vi "BEditor-PopoulateVIHelp.vi"(7 "Reference":variant, 8 "Error in":errorcluster caption="Error in (no error)", 9 "Option":variant, 11 "Entry":string) -> (0 "Error out":errorcluster)   [LabVIEW 2017, in "csmdoc.lvlib"]
uses:
  _Typedef/DocElement.ctl
  csmdoc.lvlib
  Communicable State Machine.lvlib
  _Shared/CSM Shared.lvlib
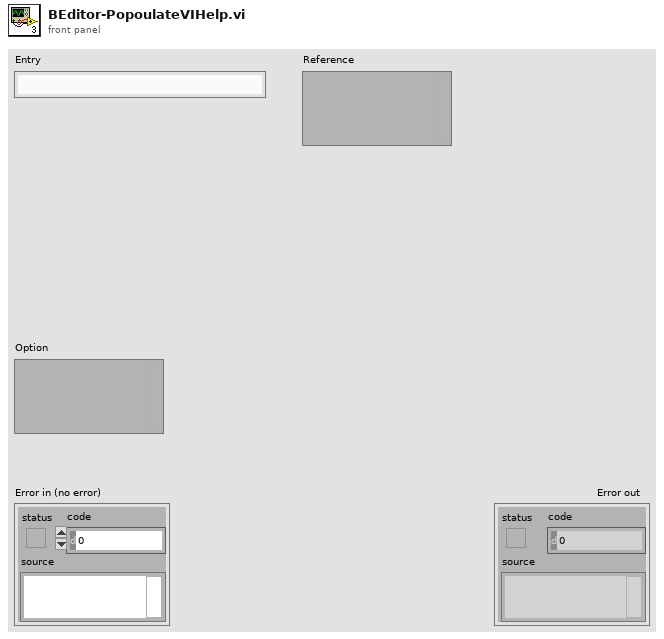
[diagram p1: front panel]
types:
  T1 = typedef "csmdoc.lvlib/DocElement.ctl" = cluster{"ID":string, "Content":string[], "SubIDs":string[], "Path":string[]}
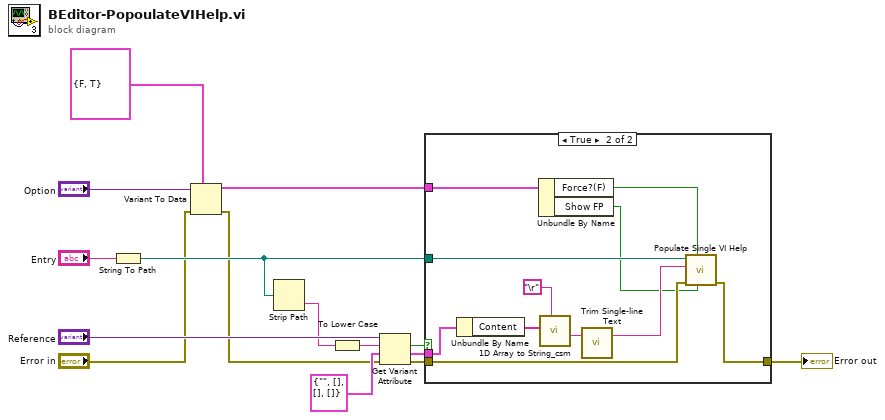
[diagram p0: block diagram]
diagram:
  n1 = String To Path(string="Entry") -> (path=w6:path)
  n2 = Variant To Data(error in="Error in", type=cluster{"Force?(F)":bool, "Show FP":bool} {"Force?(F)"=FALSE, "Show FP"=TRUE}, Variant="Option") -> (data=w1:cluster{"Force?(F)":bool, "Show FP":bool}, error out=w2:errorcluster)
  n3 = Strip Path(path=w6) -> (name=w13:string)  [unwired: 1 out]
  n4 = To Lower Case(string=w13) -> (all lower case string=w9:string)
  n5 = Get Variant Attribute(Variant="Reference", name=w9, default value (empty Variant)=T1 {"ID"="", "Content"=[], "SubIDs"=[], "Path"=[]} ("Cluster"), error in=w2) -> (found=w12:bool, value=w10:T1, error out=w11:errorcluster)  [unwired: 1 out]
  n6 = case shown="True" w12 {
    tunnel: w6 -> [_ w27]
    tunnel: w11 -> [w16 w26]
    tunnel: [w16 w25] -> w7
    tunnel: w10 -> [_ w21]
    tunnel: w1 -> [_ w19]
    frame False {
    }
    frame True {
      n7 = Unbundle By Name(w21) -> ("Content"=w24:string[])
      n8 = Unbundle By Name(w19) -> ("Force?(F)"=w18:bool, "Show FP"=w17:bool)
      n9 = call "1D Array to String_csm.vi"("delimiter (Tab)"="\r", "Array of Strings"=w24) -> ("delimited string"=w22:string)  [unwired: 9 in]
      n10 = call "Trim Single-line Text.vi"("single-line text"=w22) -> ("trimed text"=w20:string)  [unwired: 2 in]
      n11 = call "Populate Single VI Help.vi"("Show FP"=w17, "Force?(F)"=w18, "error in (no error)"=w26, "VI Description"=w20, "Path"=w27) -> ("error out"=w25:errorcluster)  [unwired: 6 in]
    }
  }
  "Error out" <- w7
